vi "Parse Anonymous Message.vi"(7 "Guess LEN Types":bool, 8 "error in (no error)":errorcluster, 11 "Buffer":u8[](array[numeric])) -> (0 "error out":errorcluster, 2 "Buffer Length":i32, 3 "Raw Message":refnum<class "Raw Message.lvclass">)   [LabVIEW 2020, in "Protobuf RAW.lvlib" / "Raw Message.lvclass"]
uses:
  Raw Message.lvclass
  VarINT Encoder/VarINT.lvclass
  E:/Labview/LV 2020/Libs/LV Protobuf Raw/Source/Protobuf RAW/Wire Type Group/Wire Type Group.lvclass
  I64 Wire/I64.lvclass
  bytes/bytes.lvclass
  E:/Labview/LV 2020/Libs/LV Protobuf Raw/Source/Protobuf RAW/LEN Encoder/LEN.lvclass
  LEN Encoder/LEN.lvclass
  I32 Encoder/I32.lvclass
  Wire Type Group/Wire Type Group.lvclass
  E:/Labview/LV 2020/Libs/LV Protobuf Raw/Source/Protobuf RAW/Tag/Basic Type.lvclass
  Raw Message.lvclass/Raw Message.ctl
  Protobuf RAW.lvlib
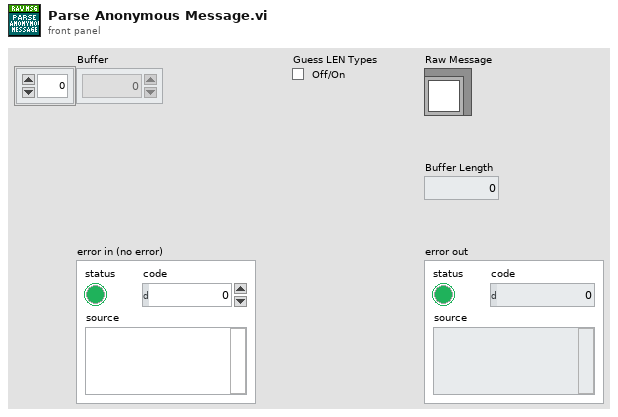
[diagram p1: front panel]
types:
  T1 = typedef "Protobuf RAW.lvlib/Wire Chunk.ctl" = cluster{"ID":u32, "Wire Type":T2, "Buffer":u8[], "length":i32}
  T2 = typedef "Protobuf RAW.lvlib/Wire Type Group.lvclass/Wire Type.ctl" = enum16{"VARINT", "I64", "LEN", "SGROUP", "EGROUP", "I32"}
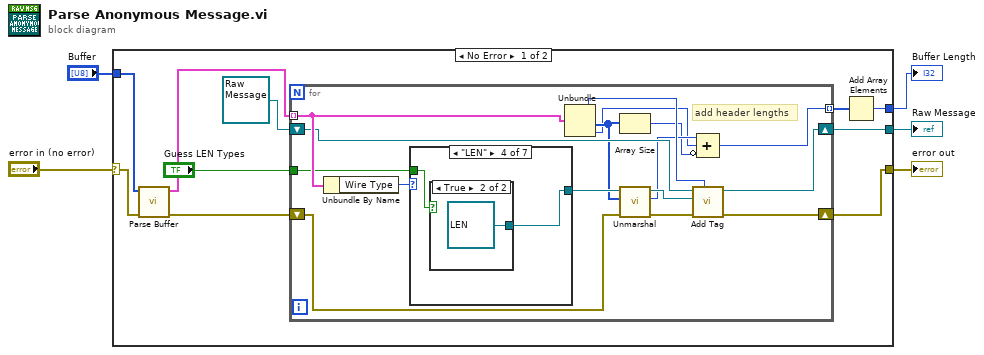
[diagram p0: block diagram]
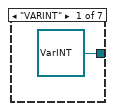
[diagram p2: hidden frame]
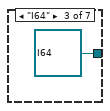
[diagram p4: hidden frame]
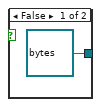
[diagram p5: hidden frame]
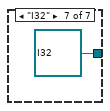
[diagram p8: hidden frame]
diagram:
  n1 = case shown="No Error" "error in (no error)" {
    selector: "error in (no error)" -> [w14 w39]
    tunnel: "Buffer" -> [w15 _]
    tunnel: [w10 _] -> w3
    tunnel: [w9 w39] -> w2
    tunnel: [w7 _] -> w1
    frame No Error {
      n2 = call "Parse Buffer.vi"("error in (no error)"=w14, "Buffer"=w15) -> ("error out"=w12:errorcluster, "Raw Fields"=w13:T1[])  [unwired: 8 in]
      n3 = for {
        tunnel: w13 -> [w29] mode=indexing
        shift-right: [w22] -> w9
        shift-left: w12 -> [w28]
        shift-right: [w26] -> w10
        shift-left: refnum<class "Raw Message.lvclass"> refnum ("Protobuf Encode.lvlib:Raw Message.lvclass") -> [w27]
        tunnel: [w18] -> w8 mode=indexing
        tunnel: "Guess LEN Types" -> [w16]
        # "add header lengths"
        n4 = Unbundle By Name(w29) -> ("Wire Type"=w31:T2)
        n5 = case shown="\"LEN\"" w31 {
          tunnel: [refnum<class "VarINT.lvclass"> refnum ("Protobuf Encode.lvlib:VarINT.lvclass") _ refnum<class "I64.lvclass"> refnum ("Protobuf Encode.lvlib:I64.lvclass") w35 _ _ refnum<class "I32.lvclass"> refnum ("Protobuf Encode.lvlib:I32.lvclass")] -> w30
          tunnel: w16 -> [_ _ _ w34 _ _ _]
          frame "VARINT" {
          }
          frame Default {
          }
          frame "I64" {
          }
          frame "LEN" {
            n6 = case shown="True" w34 {
              tunnel: [refnum<class "bytes.lvclass"> refnum ("Protobuf Encode.lvlib:LEN.lvclass") refnum<class "LEN.lvclass"> refnum ("Protobuf RAW.lvlib:LEN.lvclass")] -> w35
              frame False {
              }
              frame True {
              }
            }
          }
          frame "SGROUP" {
          }
          frame "EGROUP" {
          }
          frame "I32" {
          }
        }
        n7 = Unbundle(w29) -> ("ID"=w24:u32, "Buffer"=w20:u8[], "length"=w19:i32)  [unwired: 1 out]
        n8 = Array Size(array=w20) -> (size(s)=w17:i32)
        n9 = call-dynamic "Unmarshal.vi"("error in (no error)"=w28, "Buffer"=w20, "Type Serializer in"=w30) -> ("error out"=w23:errorcluster, "Buffer Count"=w21:i32, "Type Serializer out"=w25:refnum<class "Wire Type Group.lvclass">)  [unwired: 6 in]
        n10 = call-dynamic "Add Tag.vi"("ID"=w24, "error in (no error)"=w23, "Tag Value"=w25, "Message in"=w27) -> ("error out"=w22:errorcluster, "Message out"=w26:refnum<class "Raw Message.lvclass">)  [unwired: 6 in]
        n11 = Compound Arithmetic op=ADD(w21, w19, invert w17) -> (w18:i32)
      }
      n12 = Add Array Elements(numeric array=w8) -> (sum=w7:i32)
    }
    frame Error {
    }
  }
  "Raw Message" <- w3
  "error out" <- w2
  "Buffer Length" <- w1
